vi "SubX.vi"() -> ()   [LabVIEW 2013]
panel:
  out "32bit integer":i32
  in  "X":refnum<user-event>
  in  "stop":bool
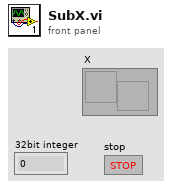
[diagram p1: front panel]
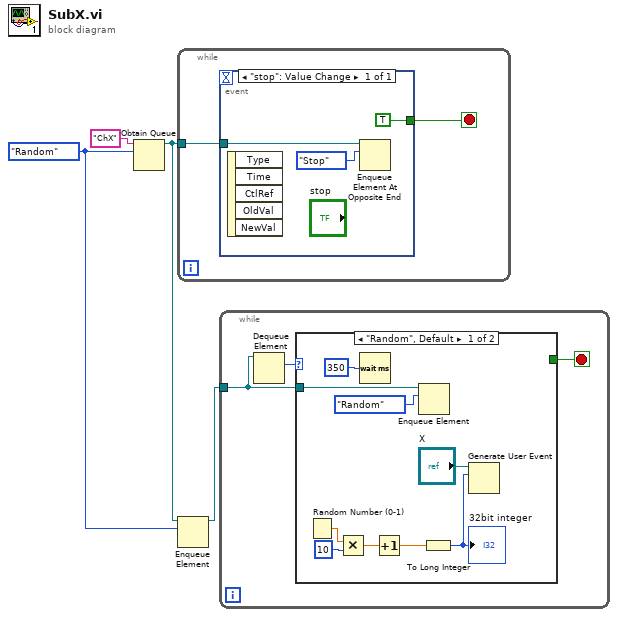
[diagram p0: block diagram]
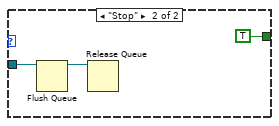
[diagram p2: hidden frame]
diagram:
  w2 = enum16{"Random", "Stop"}."Random" ("Enum")
  n1 = Obtain Queue(name (unnamed)="ChX", element data type=w2) -> (queue out=w4:refnum<queue>)  [unwired: 3 in, 2 out]
  n2 = while {
    tunnel: w4 -> [w6]
    stop <- w5 stop-if-true
    n3 = event shown="[0] \"stop\": Value Change" {
      selector: _ -> [_]
      dyn-events: _ -> [_]
      timeout: _ -> [_]
      tunnel: w6 -> [w9]
      tunnel: [TRUE] -> w5
      event "stop": Value Change {
        n4 = event-data() -> ()  [unwired: 1 in, 5 out]
        n5 = Enqueue Element At Opposite End(queue=w9, element=enum16{"Random", "Stop"}."Stop" ("Enum")) -> ()  [unwired: 2 in, 3 out]
      }
    }
  }
  n6 = Enqueue Element(queue=w4, element=w2) -> (queue out=w1:refnum<queue>)  [unwired: 2 in, 2 out]
  n7 = while {
    tunnel: w1 -> [w11]
    stop <- w10 stop-if-true
    n8 = Dequeue Element(queue=w11) -> (element=w12:enum16{"Random", "Stop"})  [unwired: 2 in, 3 out]
    n9 = case shown="\"Random\", Default" w12 {
      tunnel: [_ TRUE] -> w10
      tunnel: w11 -> [w16 w22]
      frame "Random", Default {
        n10 = Random Number (0-1)() -> (number: 0 to 1=w19:dbl)
        n11 = Multiply(x=w19, y=u32 10) -> (x*y=w14:dbl)
        n12 = Wait (ms)(milliseconds to wait=u32 350) -> ()  [unwired: 1 out]
        n13 = Increment(x=w14) -> (x+1=w13:dbl)
        n14 = Enqueue Element(queue=w16, element=enum16{"Random", "Stop"}."Random" ("Enum")) -> ()  [unwired: 2 in, 3 out]
        n15 = To Long Integer(number=w13) -> (32bit integer=w20:i32)
        "32bit integer" <- w20
        n16 = Generate User Event(user event="X", event data cluster=w20) -> ()  [unwired: 2 in, 2 out]
      }
      frame "Stop" {
        n17 = Flush Queue(queue=w22) -> (queue out=w23:refnum<queue>)  [unwired: 1 in, 2 out]
        n18 = Release Queue(queue=w23) -> ()  [unwired: 2 in, 3 out]
      }
    }
  }
